vi "Autoscale_Y_Single.vi"(11 "GraphRef":refnum<vi>) -> ()   [LabVIEW 2013]
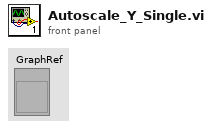
[diagram p1: front panel]
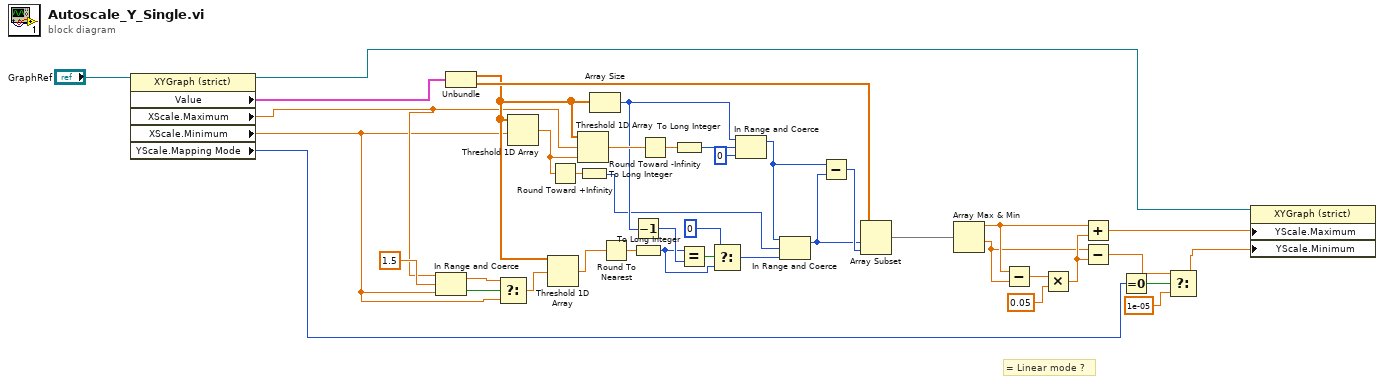
[diagram p0: block diagram]
diagram:
  # "= Linear mode ?"
  n1 = property on="Property Node" class="XYGraph (strict)"(reference="GraphRef") -> (reference out=w15:refnum<vi>, "Value"=w14:cluster{dbl[], dbl[]}, "XScale.Maximum"=w7:dbl, "XScale.Minimum"=w6:dbl, "YScale.Mapping Mode"=w2:u8)  [unwired: 1 in, 1 out]
  n2 = In Range and Coerce(upper limit=w7, x=1.5 ("threshold y"), lower limit=w6) -> (coerced(x)=w9:dbl, In Range?=w10:bool)
  n3 = Unbundle(w14) -> (w12:dbl[], w26:dbl[])
  n4 = Select(t=w9, s=w10, f=w6) -> (s? t:f=w8:dbl)
  n5 = Threshold 1D Array(2:w6, 3:w12) -> (0:w36:dbl)  [unwired: 1 in]
  n6 = Threshold 1D Array(2:w8, 3:w12) -> (0:w32:dbl)  [unwired: 1 in]
  n7 = Round Toward +Infinity(x=w36) -> (ceil(x): smallest int >= x=w34:dbl)
  n8 = Threshold 1D Array(1:w36, 2:w7, 3:w12) -> (0:w37:dbl)
  n9 = To Long Integer(number=w34) -> (32bit integer=w18:i32)
  n10 = Array Size(array=w12) -> (size(s)=w29:i32)
  n11 = Round To Nearest(number=w32) -> (nearest integer value=w30:dbl)
  n12 = Decrement(x=w29) -> (x-1=w28:i32)
  n13 = To Long Integer(number=w30) -> (32bit integer=w20:i32)
  n14 = Round Toward -Infinity(1:w37) -> (0:w24:dbl)
  n15 = To Long Integer(number=w24) -> (32bit integer=w22:i32)
  n16 = Equal?(x=w20, y=w28) -> (x = y?=w31:bool)
  n17 = Select(t=0, s=w31, f=w20) -> (s? t:f=w21:i32)
  n18 = In Range and Coerce(upper limit=w29, x=w22, lower limit=0) -> (coerced(x)=w19:i32)  [unwired: 1 out]
  n19 = In Range and Coerce(upper limit=w19, x=w18, lower limit=w21) -> (coerced(x)=w17:i32)  [unwired: 1 out]
  n20 = Subtract(x=w19, y=w17) -> (x-y=w35:i32)
  n21 = Array Subset(array=w26, index=w17, length=w35) -> (w33:dbl[])
  n22 = Array Max & Min(array=w33) -> (max value=w38:dbl, min value=w13:dbl)  [unwired: 2 out]
  n23 = Subtract(x=w38, y=w13) -> (x-y=w41:dbl)
  n24 = Multiply(x=w41, y=0.05) -> (x*y=w39:dbl)
  n25 = Add(x=w38, y=w39) -> (x+y=w25:dbl)
  n26 = Subtract(x=w13, y=w39) -> (x-y=w4:dbl)
  n27 = Equal To 0?(x=w2) -> (x = 0?=w3:bool)
  n28 = Select(t=w4, s=w3, f=1e-05) -> (s? t:f=w5:dbl)
  n29 = property on="Property Node" class="XYGraph (strict)"(reference=w15, "YScale.Maximum"=w25, "YScale.Minimum"=w5) -> ()  [unwired: 1 in, 2 out]
